vi "cluster.vi"() -> ()   [LabVIEW 2019]
uses:
  <vilib>/Math Plots/3D Math Plots/3D Surface/3D Surface XCtrl/3D Surface.xctl
  <vilib>/Math Plots/3D Math Plots/3D Surface/3D Surface Datatype/Public/Plot Helper (Vector).vi
  <vilib>/measure/NI_MABase.lvlib
  <vilib>/Math Plots/3D Math Plots/3D Surface/3D Surface Datatype/3D Surface Datatype.lvclass
panel:
  out "Array 2":T1(array[cluster]) {"MANUF. DATE" format="%<%x %.3X>T"}
  in  "Array":T1(array[cluster]) {"MANUF. DATE" format="%<%x %.3X>T"}
  out "REPORT 3":T2 {"MANUF. DATE" format="%<%x %.3X>T"}
  out "REPORT 2":T2 {"MANUF. DATE" format="%<%x %.3X>T"}
  in  "REPORT":T2 {"MANUF. DATE" format="%<%x %.3X>T"}
  out "3D Surface":refnum<class "3D Plot Datatype.lvclass">[](xcontrol)
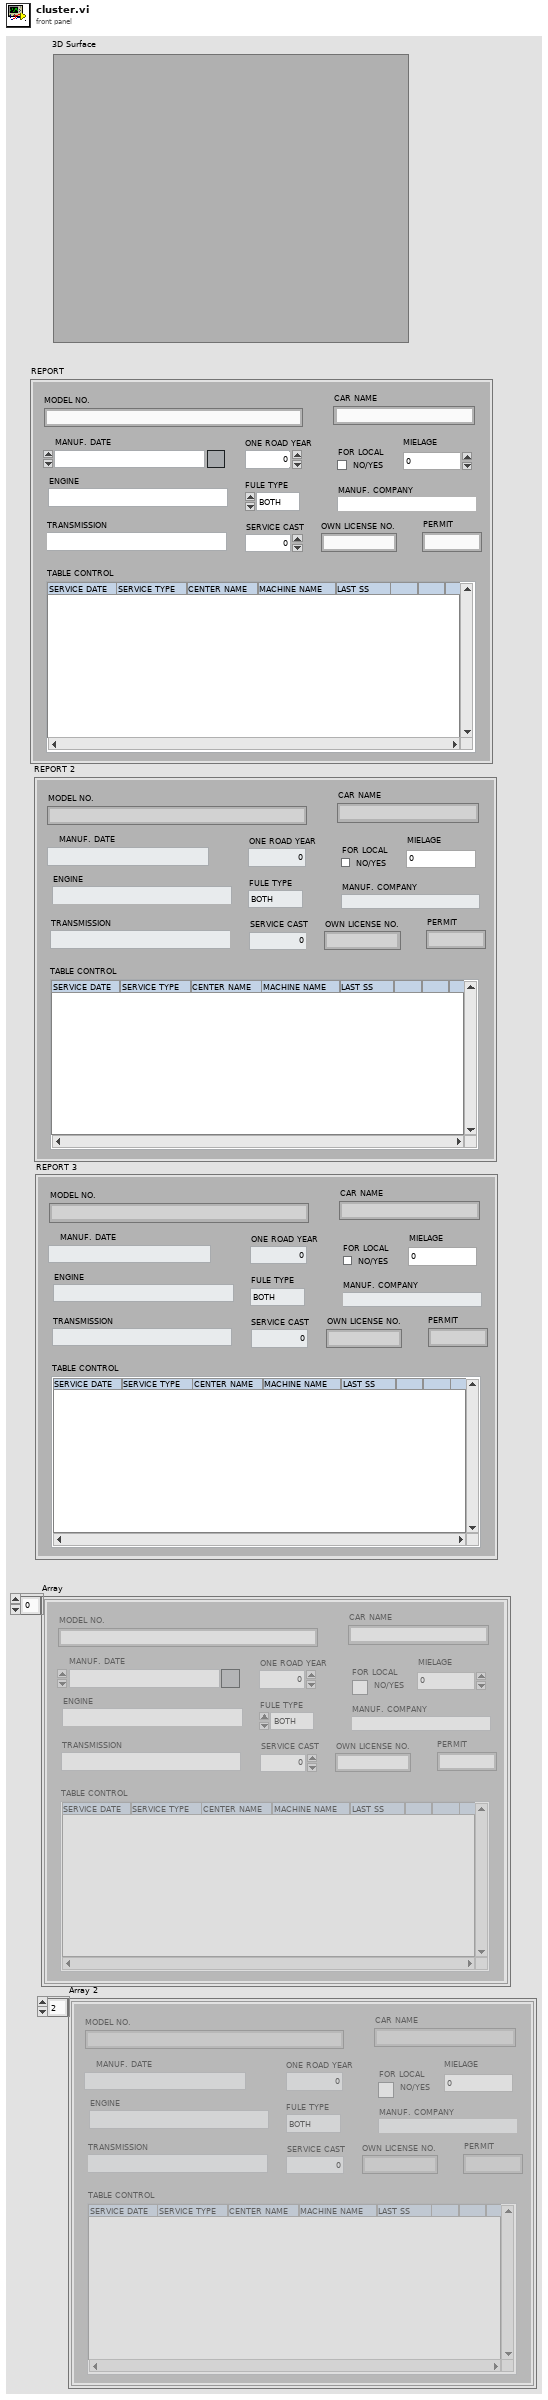
[diagram p1: front panel]
types:
  T1 = cluster{"MODEL NO.":string, "CAR NAME":string, "MANUF. DATE":timestamp, "ONE ROAD YEAR":dbl, "FOR LOCAL":bool, "MIELAGE ":dbl, "ENGINE":string, "MANUF. COMPANY":string, "TRANSMISSION":string, "TABLE CONTROL":string, "FULE TYPE":enum16{"BOTH", "PETROL", "DIESEL"}, "SERVICE CAST":dbl, "OWN LICENSE NO. ":string, "PERMIT":string}[]
  T2 = cluster{"MODEL NO.":string, "CAR NAME":string, "MANUF. DATE":timestamp, "ONE ROAD YEAR":dbl, "FOR LOCAL":bool, "MIELAGE ":dbl, "ENGINE":string, "MANUF. COMPANY":string, "TRANSMISSION":string, "TABLE CONTROL":string, "FULE TYPE":enum16{"BOTH", "PETROL", "DIESEL"}, "SERVICE CAST":dbl, "OWN LICENSE NO. ":string, "PERMIT":string}
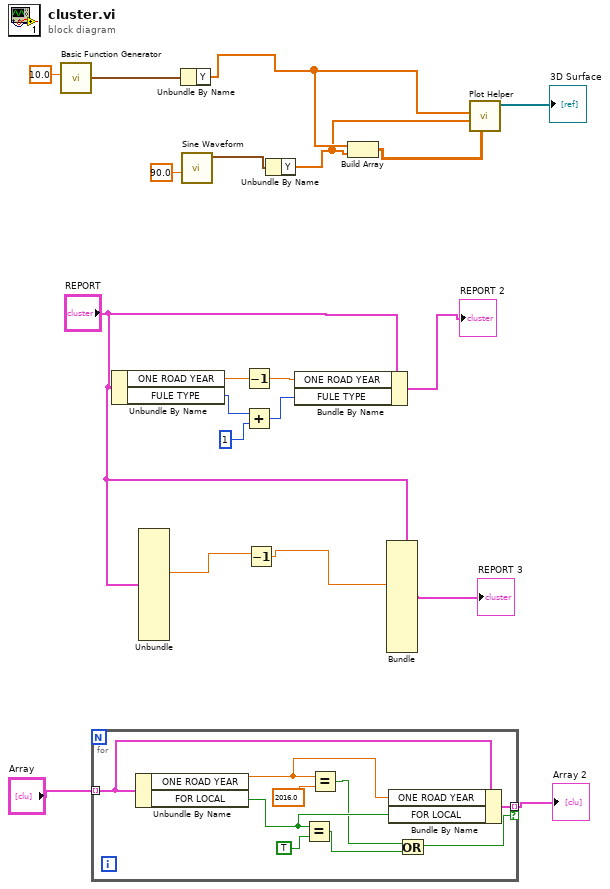
[diagram p0: block diagram]
diagram:
  n1 = call <vilib>:"Basic Function Generator.vi"("amplitude"=10.0) -> ("signal out"=w20:waveform(dbl))  [unwired: 8 in, 2 out]
  n2 = for {
    tunnel: "Array" -> [w27] mode=indexing
    tunnel: [w24] -> w1 mode=indexing if=w21
    n3 = Unbundle By Name "Unbundle By Name"(w27) -> ("ONE ROAD YEAR"=w26:dbl, "FOR LOCAL"=w25:bool)
    n4 = Equal?(x=w25, y=TRUE) -> (x = y?=w23:bool)
    n5 = Equal?(x=w26, y=2016.0) -> (x = y?=w22:bool)
    n6 = Bundle By Name(cluster=w27, "ONE ROAD YEAR"=w26, "FOR LOCAL"=w25) -> (w24:T2)
    n7 = Or(x=w22, y=w23) -> (x .or. y?=w21:bool)
  }
  "Array 2" <- w1
  n8 = Unbundle By Name "Unbundle By Name"("REPORT") -> ("ONE ROAD YEAR"=w12:dbl, "FULE TYPE"=w9:enum16{"BOTH", "PETROL", "DIESEL"})
  n9 = Unbundle "Unbundle"("REPORT") -> ("MIELAGE"=w5:dbl)  [unwired: 13 out]
  n10 = Unbundle By Name(w20) -> ("Y"=w17:dbl[])
  n11 = call <vilib>:"Sine Waveform.vi"("phase"=90.0) -> ("signal out"=w19:waveform(dbl))  [unwired: 9 in, 1 out]
  n12 = Decrement(x=w12) -> (x-1=w11:dbl)
  n13 = Add(x=w9, y=1) -> (x+y=w8:i32)
  n14 = Decrement(x=w5) -> (x-1=w4:dbl)
  n15 = Unbundle By Name(w19) -> ("Y"=w16:dbl[])
  n16 = Bundle By Name "Bundle By Name"(cluster="REPORT", "ONE ROAD YEAR"=w11, "FULE TYPE"=w8) -> (→"REPORT 2":T2)
  n17 = Build Array(w17, w16) -> (w15:dbl[][])
  n18 = Bundle "Bundle"(cluster="REPORT", "MIELAGE"=w4) -> (→"REPORT 3":T2)  [unwired: 13 in]
  n19 = call-poly <vilib>:"Plot Helper.vi"("z matrix"=w15, "y vector"=w16, "x vector"=w17) -> ("3D Plot lvclass Array out"=→"3D Surface":refnum<class "3D Plot Datatype.lvclass">[])  [unwired: 3 in, 5 out]
